vi "Sub_nonuniform_samples append_and_truncate.vi"(0 "acc in":dbl[](array[numeric]), 5 "time in":dbl[](array[numeric]), 7 "acc append":dbl[](array[numeric]), 9 "sample rate":dbl, 11 "t0":dbl, 12 "Setup Parameters":T2, 13 "Experimental Results":T1) -> (4 "acc":dbl[](array[numeric]), 6 "time out":dbl[](array[numeric]))   [LabVIEW 2019]
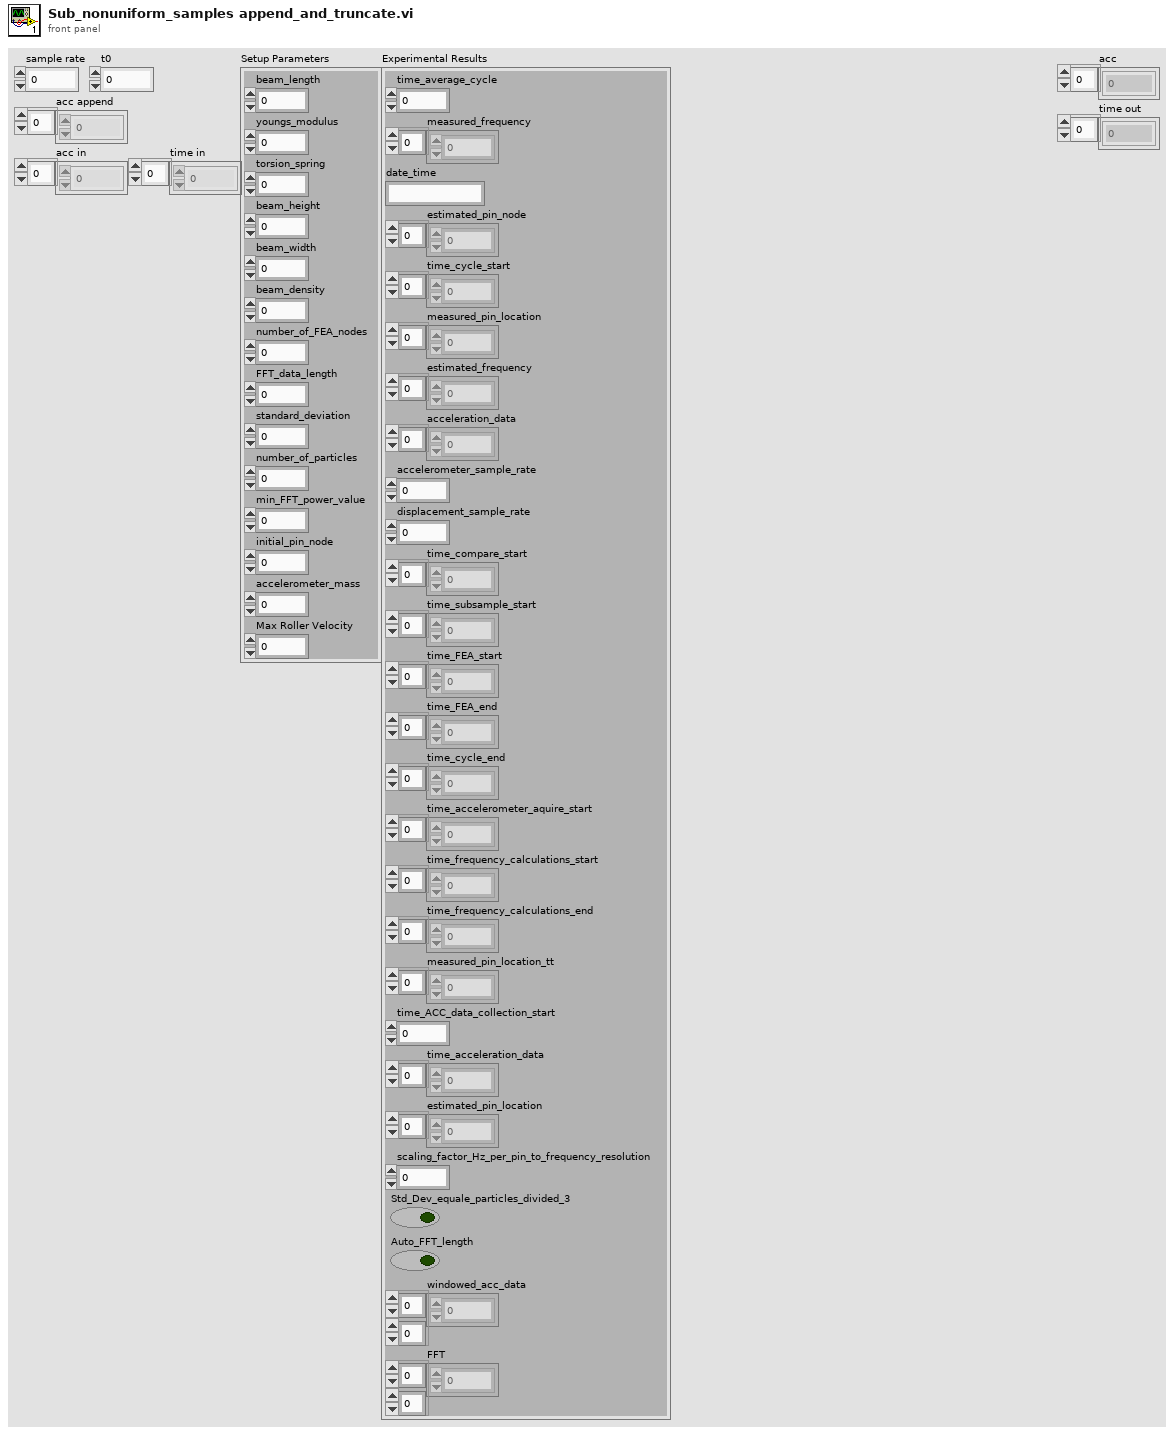
[diagram p1: front panel]
types:
  T1 = cluster{"time_average_cycle":dbl, "measured_frequency":dbl[], "date_time":string, "estimated_pin_node":i32[], "time_cycle_start":dbl[], "measured_pin_location":dbl[], "estimated_frequency":dbl[], "acceleration_data":dbl[], "accelerometer_sample_rate":dbl, "displacement_sample_rate":dbl, "time_compare_start":dbl[], "time_subsample_start":dbl[], "time_FEA_start":dbl[], "time_FEA_end":dbl[], "time_cycle_end":dbl[], "time_accelerometer_aquire_start":dbl[], "time_frequency_calculations_start":dbl[], "time_frequency_calculations_end":dbl[], "measured_pin_location_tt":dbl[], "time_ACC_data_collection_start":dbl, "time_acceleration_data":dbl[], "estimated_pin_location":dbl[], "scaling_factor_Hz_per_pin_to_frequency_resolution":dbl, "Std_Dev_equale_particles_divided_3":bool, "Auto_FFT_length":bool, "windowed_acc_data":dbl[][], "FFT":dbl[][]}
  T2 = cluster{"beam_length":dbl, "youngs_modulus":dbl, "torsion_spring":dbl, "beam_height":dbl, "beam_width":dbl, "beam_density":dbl, "number_of_FEA_nodes":i32, "FFT_data_length":i32, "standard_deviation":dbl, "number_of_particles":i32, "min_FFT_power_value":dbl, "initial_pin_node":i32, "accelerometer_mass":dbl, "Max Roller Velocity":dbl}
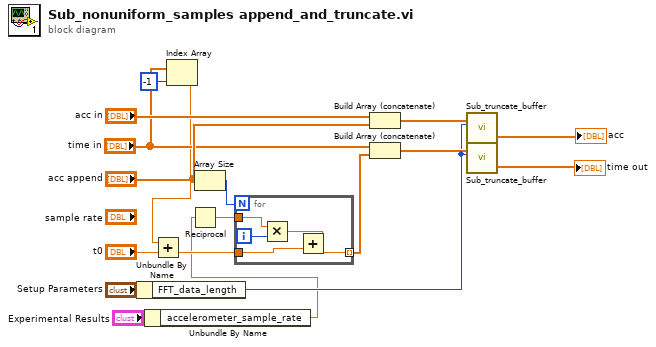
[diagram p0: block diagram]
diagram:
  n1 = Unbundle By Name("Setup Parameters") -> ("FFT_data_length"=w8:i32)
  n2 = Unbundle By Name("Experimental Results") -> ("accelerometer_sample_rate"=w1:dbl)
  n3 = Index Array(array="time in", index=-1) -> (element=w3:dbl)
  n4 = Add(x=w3, y="t0") -> (x+y=w4:dbl)
  n5 = Reciprocal(x=w1) -> (1/x=w16:dbl)
  n6 = Array Size(array="acc append") -> (size(s)=w18:i32)
  n7 = for {
    N: w18 -> [_]
    tunnel: w4 -> [w23]
    tunnel: [w21] -> w12 mode=indexing
    tunnel: w16 -> [w19]
    i -> [w22]
    n8 = Multiply(x=w19, y=w22) -> (x*y=w20:dbl)
    n9 = Add(x=w20, y=w23) -> (x+y=w21:dbl)
  }
  n10 = Build Array (concatenate)("acc in", "acc append") -> (w13:dbl[])
  n11 = Build Array (concatenate)("time in", w12) -> (w11:dbl[])
  n12 = call "Sub_truncate_buffer.vi"("array"=w13, "samples"=w8) -> ("array"=→"acc":dbl[])  [unwired: 9 in]
  n13 = call "Sub_truncate_buffer.vi"("array"=w11, "samples"=w8) -> ("array"=→"time out":dbl[])  [unwired: 9 in]
